vi "FileSelector.vi"(6 "array size":i32, 9 "index in":i32, 11 "Selection Controls":cluster{"Up":bool, "Down":bool}) -> (1 "index out":i32, 3 "isChanged":bool)   [LabVIEW 2013]
uses:
  Common Code/Change Detect Boolean.vi
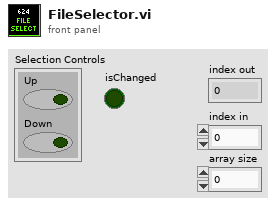
[diagram p1: front panel]
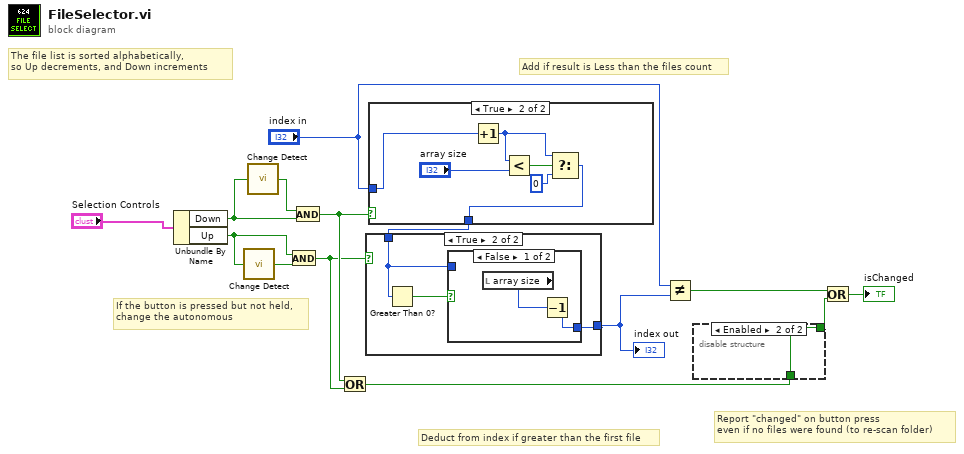
[diagram p0: block diagram]
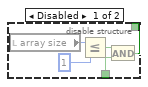
[diagram p2: hidden frame]
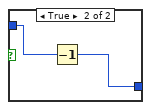
[diagram p5: hidden frame]
diagram:
  # "The file list is sorted alphabetically,\nso Up decrements, and Down increments"
  # "Report \"changed\" on button press\neven if no files were found (to re-scan folder)"
  # "If the button is pressed but not held,\nchange the autonomous"
  # "Add if result is Less than the files count"
  # "Deduct from index if greater than the first file"
  n1 = Unbundle By Name("Selection Controls") -> ("Down"=w12:bool, "Up"=w9:bool)
  n2 = call-poly "Change Detect.vi"("In"=w9) -> ("Changed?"=w10:bool)
  n3 = call-poly "Change Detect.vi"("In"=w12) -> ("Changed?"=w11:bool)
  n4 = And(x=w9, y=w10) -> (x .and. y?=w1:bool)
  n5 = And(x=w11, y=w12) -> (x .and. y?=w2:bool)
  n6 = Or(x=w2, y=w1) -> (x .or. y?=w3:bool)
  n7 = case shown="True" w2 {
    tunnel: "index in" -> [w15 w18]
    tunnel: [w15 w19] -> w14
    frame False {
    }
    frame True {
      n8 = Increment(x=w18) -> (x+1=w20:i32)
      n9 = Less?(x=w20, y="array size") -> (x < y?=w21:bool)
      n10 = Select(t=w20, s=w21, f=0) -> (s? t:f=w19:i32)
    }
  }
  n11 = case shown="True" w1 {
    tunnel: w14 -> [w22 w24]
    tunnel: [w22 w23] -> w13
    frame False {
    }
    frame True {
      n12 = Greater Than 0?(x=w24) -> (x > 0?=w25:bool)
      n13 = case shown="False" w25 {
        tunnel: w24 -> [_ w29]
        tunnel: [w26 w28] -> w23
        frame False {
          n14 = local read "array size"() -> (w27:i32)
          n15 = Decrement(x=w27) -> (x-1=w26:i32)
        }
        frame True {
          n16 = Decrement(x=w29) -> (x-1=w28:i32)
        }
      }
    }
  }
  "index out" <- w13
  n17 = Not Equal?(x="index in", y=w13) -> (x != y?=w7:bool)
  n18 = disable-structure shown="Enabled" {
    disable-tunnel: [w33 w35] -> w5
    disable-tunnel: w3 -> [w32 w35]
    frame Disabled {
      n19 = local read "array size"() -> (w30:i32)
      n20 = Less Or Equal?(x=w30, y=1) -> (x <= y?=w34:bool)
      n21 = And(x=w34, y=w32) -> (x .and. y?=w33:bool)
    }
    frame Enabled {
    }
  }
  n22 = Or(x=w7, y=w5) -> (x .or. y?=→"isChanged":bool)
